vi "Rectangel ContainsInBound.vi"(1 "point2D":T2 {"y" format="%.2f"; "x" format="%.2f"}, 2 "bounds":T1 {"height" format="%.2f"; "width" format="%.2f"; "y" format="%.2f"; "x" format="%.2f"}, 3 "AdditionalMargin":i32, 5 "error in (no error)":errorcluster) -> (15 "contains":bool, 19 "error out":errorcluster)   [LabVIEW 2020]
doc: "contains"
uses:
  <resource>/Framework/Providers/Open_GDS/UML/General/Point/Point Point2D.ctl
  <resource>/Framework/Providers/Open_GDS/UML/General/Rectangle/Rectangle Rectangle2D.ctl
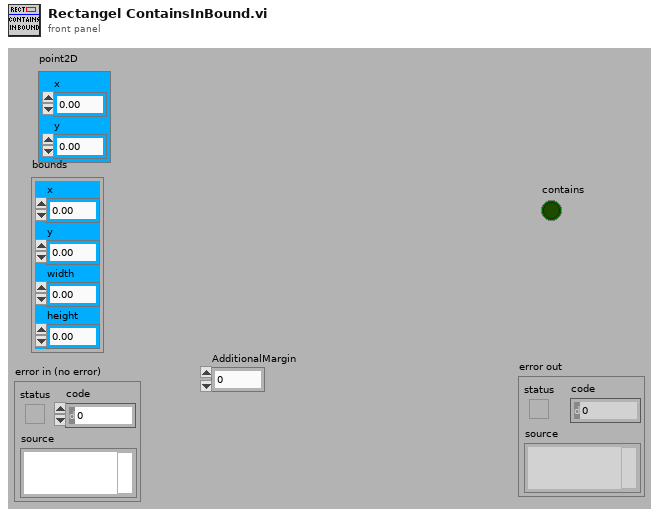
[diagram p1: front panel]
types:
  T1 = typedef "Rectangle Rectangle2D.ctl" = cluster{"x":dbl, "y":dbl, "width":dbl, "height":dbl}
  T2 = typedef "Point Point2D.ctl" = cluster{"x":dbl, "y":dbl}
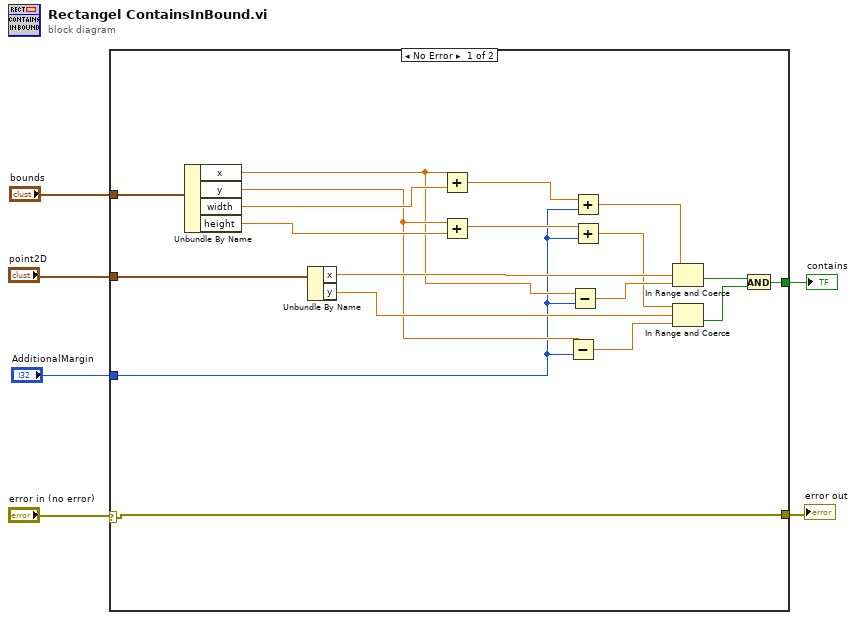
[diagram p0: block diagram]
diagram:
  n1 = case shown="No Error" "error in (no error)" {
    selector: "error in (no error)" -> [w17 w26]
    tunnel: [w17 w26] -> w6
    tunnel: "point2D" -> [w25 _]
    tunnel: [w24 _] -> w3
    tunnel: "bounds" -> [w19 _]
    tunnel: "AdditionalMargin" -> [w8 _]
    frame No Error {
      n2 = Unbundle By Name(w19) -> ("x"=w13:dbl, "y"=w15:dbl, "width"=w18:dbl, "height"=w16:dbl)
      n3 = Unbundle By Name(w25) -> ("x"=w23:dbl, "y"=w22:dbl)
      n4 = Add(x=w13, y=w18) -> (x+y=w11:dbl)
      n5 = Add(x=w15, y=w16) -> (x+y=w10:dbl)
      n6 = Subtract(x=w15, y=w8) -> (x-y=w14:dbl)
      n7 = Subtract(x=w13, y=w8) -> (x-y=w12:dbl)
      n8 = Add(x=w11, y=w8) -> (x+y=w9:dbl)
      n9 = Add(x=w10, y=w8) -> (x+y=w7:dbl)
      n10 = In Range and Coerce(upper limit=w9, x=w23, lower limit=w12) -> (In Range?=w21:bool)  [unwired: 1 out]
      n11 = In Range and Coerce(upper limit=w7, x=w22, lower limit=w14) -> (In Range?=w20:bool)  [unwired: 1 out]
      n12 = And(x=w21, y=w20) -> (x .and. y?=w24:bool)
    }
    frame Error {
    }
  }
  "error out" <- w6
  "contains" <- w3
